vi "AWS-S3-UploadFile.vi"(0 "Mini AWS S3 API":refnum<class "AWS-S3-MiniAPI.lvclass">, 5 "Object Key":string, 7 "Object Bucket":string, 9 "Source Filepath (Local)":path, 11 "error in":errorcluster) -> (4 "Mini AWS S3 API out":refnum<class "AWS-S3-MiniAPI.lvclass">, 8 "Object Download URL":string, 15 "error out":errorcluster)   [LabVIEW 2012, in "AWS-S3-MiniAPI.lvclass"]
uses:
  AWS-S3-MiniAPI.lvclass
  AWS-S3-MiniAPI.lvclass/AWS-S3-MiniAPI.ctl
  C:/Users/Jack/cla-2013-deployment-automation-and-release-engineering-in-labview/Deployment/AWS-SDK/AWSSDK.dll
  AWS-SDK/AWSSDK.dll
panel:
  # "Inputs"
  # "Outputs"
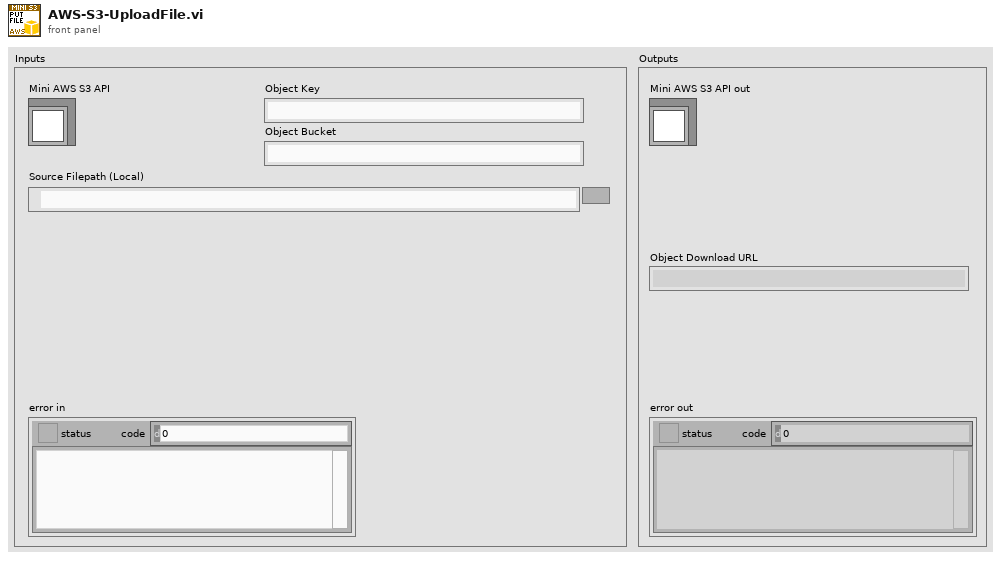
[diagram p1: front panel]
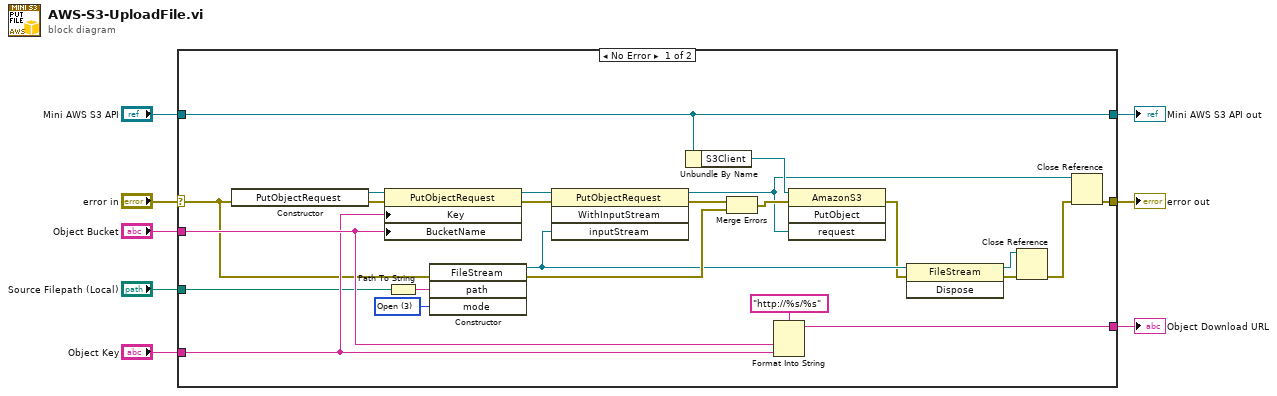
[diagram p0: block diagram]
diagram:
  n1 = case shown="No Error" "error in" {
    selector: "error in" -> [w16 w34]
    tunnel: [w9 w34] -> w8
    tunnel: [w20 w33] -> w6
    tunnel: "Mini AWS S3 API" -> [w20 w33]
    tunnel: "Source Filepath (Local)" -> [w22 _]
    tunnel: "Object Key" -> [w24 _]
    tunnel: "Object Bucket" -> [w25 _]
    tunnel: [w23 _] -> w1
    frame No Error {
      w27 = 3 items=["CreateNew"=1, "Create"=2, "Open"=3, "OpenOrCreate"=4, "Truncate"=5, "Append"=6] ("mode")
      n2 = constructor class="PutObjectRequest"(error in=w16) -> (reference out=w30:refnum<k24>, error out=w31:errorcluster)  [unwired: 2 in, 1 out]
      n3 = property class="PutObjectRequest"(reference=w30, error in=w31, "Key"=w24, "BucketName"=w25) -> (reference out=w18:refnum<k24>, error out=w17:errorcluster)
      n4 = Path To String(path=w22) -> (string=w28:string)
      n5 = constructor class="FileStream"(error in=w16, "path"=w28, "mode"=w27) -> (reference out=w15:refnum<k24>, error out=w32:errorcluster)  [unwired: 2 in, 3 out]
      n6 = invoke class="PutObjectRequest" method="WithInputStream"(reference=w18, error in=w17, "inputStream"=w15) -> (reference out=w11:refnum<k24>, error out=w29:errorcluster)  [unwired: 1 in, 2 out]
      n7 = Unbundle By Name(w20) -> ("S3Client"=w21:refnum<k24>)
      n8 = Merge Errors(w29, w32) -> (w19:errorcluster)
      n9 = Format Into String(format string="http://%s/%s", w25, w24) -> (resulting string=w23:string)  [unwired: 2 in, 1 out]
      n10 = invoke class="AmazonS3" method="PutObject"(reference=w21, error in=w19, "request"=w11) -> (error out=w14:errorcluster)  [unwired: 1 in, 3 out]
      n11 = invoke class="FileStream" method="Dispose"(reference=w15, error in=w14) -> (reference out=w13:refnum<k24>, error out=w12:errorcluster)  [unwired: 1 in, 1 out]
      n12 = Close Reference(reference=w13, error in (no error)=w12) -> (error out=w10:errorcluster)
      n13 = Close Reference(reference=w11, error in (no error)=w10) -> (error out=w9:errorcluster)
    }
    frame Error {
    }
  }
  "error out" <- w8
  "Mini AWS S3 API out" <- w6
  "Object Download URL" <- w1
